vi "Postprocessing aktiv.vi"() -> (1 "automatisch out":T1, 3 "postprocess":bool)   [LabVIEW 2020, in "Linearisierung v2.lvlib"]
uses:
  Linearisierung v2.lvlib
  SpanEinstellungen/Aktion FGV SpanEinstellungen.ctl
  SpanEinstellungen/SpanEinstellungen.lvlib
  Seiten/System Einstellungen V2/Konfig Gasflasche.ctl
  Seiten/System Einstellungen V2/System Einstellungen V2.lvlib
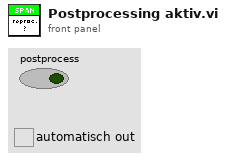
[diagram p1: front panel]
types:
  T1 = typedef "System Einstellungen V2.lvlib/Konfig Gasflasche.ctl" = bool
  T2 = typedef "Linearisierung v2.lvlib/SpanEinstellungen.lvlib/Aktion FGV SpanEinstellungen.ctl" = enum16{"lesen", "schreiben", "laden", "speichern", "RegisterRef", "automatisch", "init", "PDF Params", "Punkte umkehren"}
  T3 = typedef "Linearisierung v2.lvlib/SpanEinstellungen.lvlib/SpanInletCluster.ctl" = cluster{"Span Inlet Active":T1, "Analysator":T4, "Konfig Gasflasche":T1, "Gasflasche":T5, "Gasflaschen Nr.:":string, "Ablaufdatum":timestamp, "Komponenten":T6, "Zeitdauer Stufen":sgl, "Max Fehler":sgl, "Anzahl Stufen":sgl, "Trägergas":T10, "zusätzliche Zeitdauer Erster Punkt":sgl}
  T4 = typedef "System Einstellungen V2.lvlib/Analysatoren.ctl" = string
  T5 = typedef "System Einstellungen V2.lvlib/Gasflasche Auswahl.ctl" = u16
  T6 = typedef "Linearisierung v2.lvlib/SpanEinstellungen.lvlib/Komponentencluster mit Formel.ctl" = cluster{"Komponente 1":T7, "Komponente 2":T7, "Komponente 3":T7, "Komponente 4":T7, "Komponente 5":T7}
  T7 = typedef "Linearisierung v2.lvlib/SpanEinstellungen.lvlib/Komponentenauswahl mit Formel.ctl" = cluster{"Komponente:":u16, "Summenformel":T8, "Konzentration IST":dbl, "Einheit":T9, "Genauigkeit":dbl}
  T8 = typedef "String - Eingabefeld.ctl" = string
  T9 = typedef "Linearisierung v2.lvlib/SpanEinstellungen.lvlib/Einheit.ctl" = enum16{"ppm", "%"}
  T10 = typedef "System Einstellungen V2.lvlib/Traegergas.ctl" = string
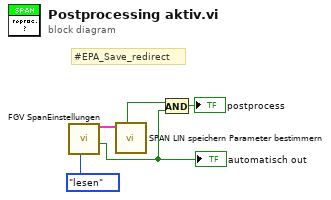
[diagram p0: block diagram]
diagram:
  # "#EPA_Save_redirect"
  n1 = call "FGV SpanEinstellungen.vi"("Aktion"=Aktion_FGV_SpanEinstellungen."lesen") -> ("automatisch out"=w1:T1, "SpanInletClusterArray out"=w3:T3[])  [unwired: 6 in, 3 out]
  "automatisch out" <- w1
  n2 = call "SPAN LIN speichern Parameter bestimmern.vi"("SpanInletClusterArray out (Eingang)"=w3) -> ("postprocess"=w5:bool)  [unwired: 2 in, 8 out]
  n3 = And(x=w5, y=w1) -> (x .and. y?=→"postprocess":T1)
